vi "Initialize Actor.vi"(7 "Host Name":string, 8 "error in (no error)":errorcluster, 9 "Actor Name":string, 10 "Message Broker Interface":refnum<class "Message Broker Interface.lvclass">, 11 "Car Wash Station Sequencer in":refnum<class "Car Wash Station Sequencer.lvclass">) -> (0 "error out":errorcluster, 3 "Car Wash Station Sequencer out":refnum<class "Car Wash Station Sequencer.lvclass">)   [LabVIEW 2016, in "CLD Exam - Car Wash.lvlib" / "Car Wash Station Sequencer.lvclass"]
doc: "--\nCopyright © 2017 Composed SystemsI All rights reserved.\n\nAuthor: Jon McBee <jon.mcbee@composed.io>\n\nThis library is provided \"AS IS\" ,WITHOUT WARRANTIES OR\nCONDITIONS OF ANY KIND, either express or implied.\n\nComposed Systems -- composed.io\n\nStream 0.0.1.1\nJon McBee - Composed Systems\nCopyright (c) 2017, Composed Systems"
uses:
  Car Wash Station Sequencer.lvclass
  Mediator/Classes/Message Broker Interface/Message Broker Interface.lvclass
  Car Wash Station Sequencer.lvclass/Car Wash Station Sequencer.ctl
  Mediator/Classes/Message Transport Event/Message Transport Event.lvclass
  D:/Repos/Stream/software/Mediator/Classes/Message Transport Interface/Message Transport Interface.lvclass
  Mediator/Classes/Mediated Synchronous Actor/Mediated Synchronous Actor.lvclass
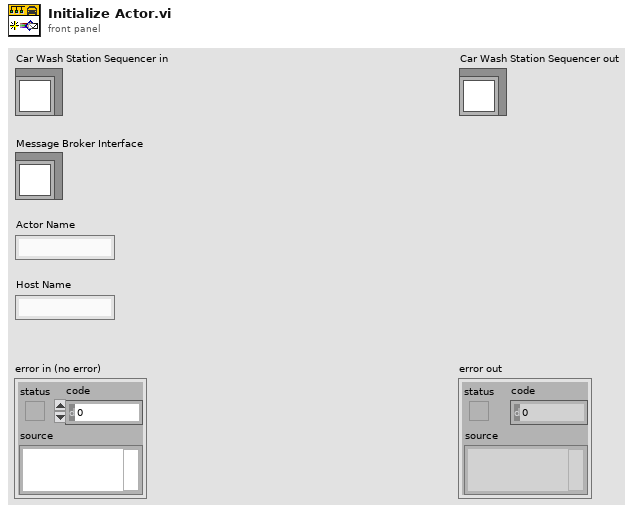
[diagram p1: front panel]
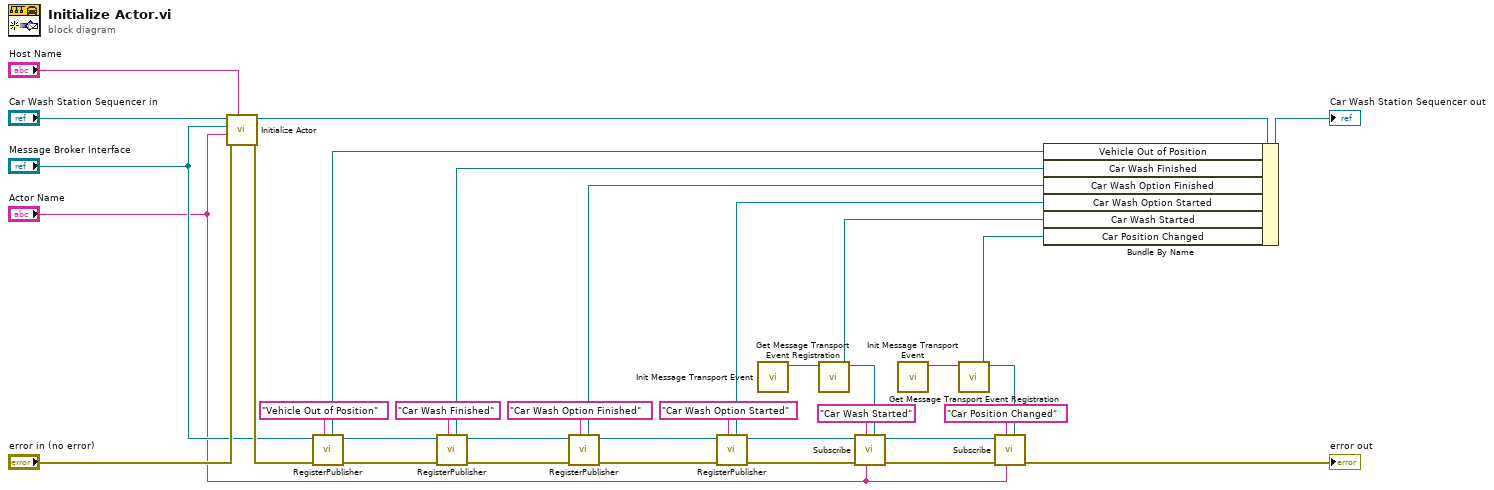
[diagram p0: block diagram]
diagram:
  n1 = call-parent "Initialize Actor.vi"("Host Name"="Host Name", "error in (no error)"="error in (no error)", "Actor Name"="Actor Name", "Message Broker Interface"="Message Broker Interface", "Mediated Synchronous Actor in"="Car Wash Station Sequencer in") -> ("error out"=w29:errorcluster, "Mediated Synchronous Actor out"=w32:refnum<class "Car Wash Station Sequencer.lvclass">)  [unwired: 5 in]
  n2 = call-dynamic "RegisterPublisher.vi"("Topic Name"="Vehicle Out of Position", "error in (no error)"=w29, "Message Broker Interface in"="Message Broker Interface") -> ("error out"=w24:errorcluster, "Message Broker Interface out"=w25:refnum<class "Message Broker Interface.lvclass">, "Transport"=w27:refnum<class "Message Transport Queue.lvclass">)  [unwired: 4 in, 2 out]
  n3 = call-dynamic "RegisterPublisher.vi"("Topic Name"="Car Wash Finished", "error in (no error)"=w24, "Message Broker Interface in"=w25) -> ("error out"=w20:errorcluster, "Message Broker Interface out"=w21:refnum<class "Message Broker Interface.lvclass">, "Transport"=w23:refnum<class "Message Transport Queue.lvclass">)  [unwired: 4 in, 2 out]
  n4 = call-dynamic "RegisterPublisher.vi"("Topic Name"="Car Wash Option Finished", "error in (no error)"=w20, "Message Broker Interface in"=w21) -> ("error out"=w16:errorcluster, "Message Broker Interface out"=w17:refnum<class "Message Broker Interface.lvclass">, "Transport"=w19:refnum<class "Message Transport Queue.lvclass">)  [unwired: 4 in, 2 out]
  n5 = call-dynamic "RegisterPublisher.vi"("Topic Name"="Car Wash Option Started", "error in (no error)"=w16, "Message Broker Interface in"=w17) -> ("error out"=w5:errorcluster, "Message Broker Interface out"=w6:refnum<class "Message Broker Interface.lvclass">, "Transport"=w15:refnum<class "Message Transport Queue.lvclass">)  [unwired: 4 in, 2 out]
  n6 = call "Init Message Transport Event.vi"() -> ("Message Transport Event out"=w14:refnum<class "Message Transport Event.lvclass">)  [unwired: 10 in, 1 out]
  n7 = call "Get Message Transport Event Registration.vi"("Message Transport Event in"=w14) -> ("Event Registration Refnum"=w3:refnum<event-registration>, "Message Transport Event out"=w13:refnum<class "Message Transport Event.lvclass">)  [unwired: 7 in, 2 out]
  n8 = call-dynamic "Subscribe.vi"("Message Transport Interface"=w13, "Subscriber Name"="Actor Name", "Topic Name"="Car Wash Started", "error in (no error)"=w5, "Message Broker Interface in"=w6) -> ("error out"=w8:errorcluster, "Message Broker Interface out"=w7:refnum<class "Message Broker Interface.lvclass">)  [unwired: 4 in, 1 out]
  n9 = call "Init Message Transport Event.vi"() -> ("Message Transport Event out"=w9:refnum<class "Message Transport Event.lvclass">)  [unwired: 10 in, 1 out]
  n10 = call "Get Message Transport Event Registration.vi"("Message Transport Event in"=w9) -> ("Event Registration Refnum"=w2:refnum<event-registration>, "Message Transport Event out"=w10:refnum<class "Message Transport Event.lvclass">)  [unwired: 7 in, 2 out]
  n11 = call-dynamic "Subscribe.vi"("Message Transport Interface"=w10, "Subscriber Name"="Actor Name", "Topic Name"="Car Position Changed", "error in (no error)"=w8, "Message Broker Interface in"=w7) -> ("error out"=→"error out":errorcluster)  [unwired: 4 in, 2 out]
  n12 = Bundle By Name(cluster=w32, "Vehicle Out of Position"=w27, "Car Wash Finished"=w23, "Car Wash Option Finished"=w19, "Car Wash Option Started"=w15, "Car Wash Started"=w3, "Car Position Changed"=w2) -> (→"Car Wash Station Sequencer out":refnum<class "Car Wash Station Sequencer.lvclass">)
